vi "VarFLS.vi"(1 "D":dbl, 2 "B":dbl, 3 "B=0":bool, 4 "D=0":bool) -> (0 "FLS":dbl)   [LabVIEW 2012]
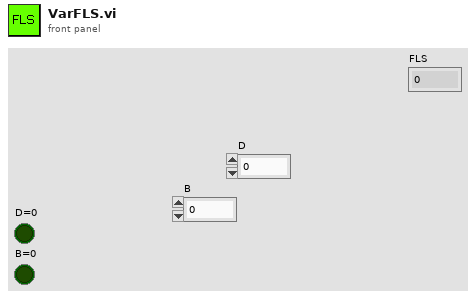
[diagram p1: front panel]
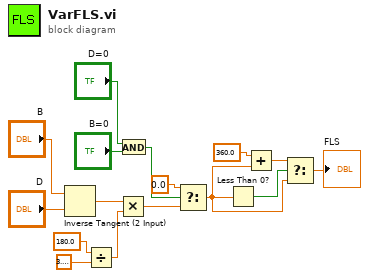
[diagram p0: block diagram]
diagram:
  n1 = Inverse Tangent (2 Input)(1:"D", 2:"B") -> (0:w7:dbl)
  n2 = Divide(x=180.0, y=3.141592653589793) -> (x/y=w8:dbl)
  n3 = Multiply(x=w7, y=w8) -> (x*y=w6:dbl)
  n4 = And(x="D=0", y="B=0") -> (x .and. y?=w14:bool)
  n5 = Select(t=0.0, s=w14, f=w6) -> (s? t:f=w2:dbl)
  n6 = Less Than 0?(x=w2) -> (x < 0?=w5:bool)
  n7 = Add(x=360.0, y=w2) -> (x+y=w4:dbl)
  n8 = Select(t=w4, s=w5, f=w2) -> (s? t:f=→"FLS":dbl)
